vi "ValueSignalLatchBooleanArray.vi"(0 "VI Reference In":refnum<vi>, 5 "Control Path":string[](array[string]), 11 "error in":errorcluster) -> (4 "VI Reference Out":refnum<vi>, 15 "error out":errorcluster)   [LabVIEW 2016, in "Drona.lvlib" / "ControlValue.lvlib"]
doc: "Triggers the latch boolean by keyboard simulation.\n\nThe path of the control should be given in the successive index of the array"
uses:
  ControlValue.lvlib
  KeyBoardSimulation/typedef/VirtualKey.ctl
  VI/MakeVIFrontMost.vi
  Get/GetControlRef/GetControlRef.lvlib
  Drona.lvlib
  KeyBoardSimulation/KeyboardSimulation.lvlib
  VI/VI.lvlib
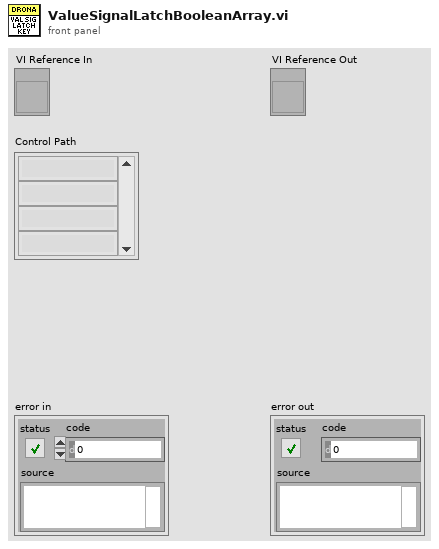
[diagram p1: front panel]
types:
  T1 = typedef "Drona.lvlib/KeyboardSimulation.lvlib/VirtualKey.ctl" = u8
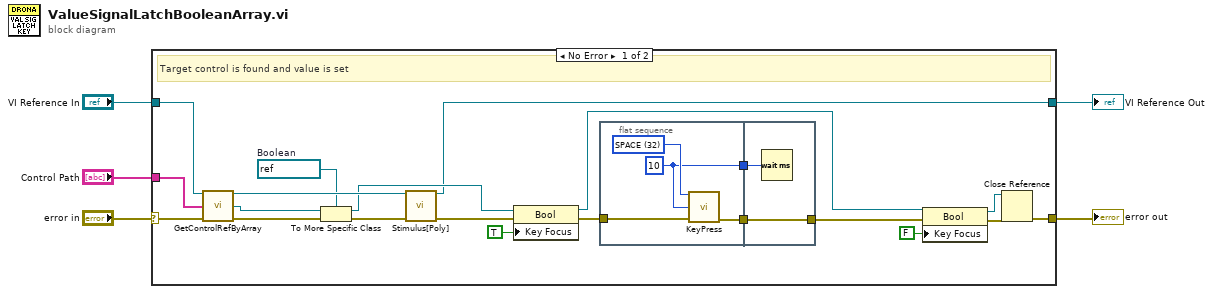
[diagram p0: block diagram]
diagram:
  n1 = case shown="No Error" "error in" {
    selector: "error in" -> [w26 w34]
    tunnel: "Control Path" -> [w24 _]
    tunnel: "VI Reference In" -> [w23 w33]
    tunnel: [w14 w33] -> w2
    tunnel: [w22 w34] -> w1
    frame No Error {
      w18 = refnum<vi> refnum  # Boolean
      # "Target control is found and value is set"
      n2 = call "GetControlRefByArray.vi"("VI Reference In"=w23, "Control Path"=w24, "error In"=w26) -> ("VI Reference Out"=w20:refnum<vi>, "Ctl Refnum"=w21:refnum<vi>, "error out"=w25:errorcluster)  [unwired: 10 in]
      n3 = To More Specific Class(target class=w18, reference=w21, error in=w25) -> (specific class reference=w17:refnum<vi>, error out=w19:errorcluster)
      n4 = call-poly "Stimulus[Poly].vi"("VI Reference In"=w20, "error in"=w19) -> ("VI Reference Out"=w14:refnum<vi>, "error out"=w16:errorcluster)  [unwired: 12 in]
      n5 = property class="Bool"(reference=w17, error in=w16, "Key Focus"=TRUE) -> (reference out=w12:refnum<vi>, error out=w9:errorcluster)
      n6 = flat-sequence {
        tunnel: w9 -> [w30]
        tunnel: [w29] -> w7
        tunnel: [w27] -> w6
        tunnel: [w32] -> w8
        tunnel: w7 -> [w32]
        tunnel: w6 -> [w31]
        frame #0 {
          w27 = u32 10 ("Millis")
          w28 = T1 32 items=["LBUTTON"=1, "RBUTTON"=2, "CANCEL"=3, "MBUTTON"=4, "BACKSPACE"=8, "TAB"=9, "CLEAR"=12, "ENTER"=13, "SHIFT"=16, "CTRL"=17, "ALT"=18, "PAUSE"=19, "CAPITAL"=20, "ESCAPE"=27, "SPACE"=32, "PAGEUP"=33, "PAGEDOWN"=34, "END"=35, "HOME"=36, "LEFTARROW"=37, "UPARROW"=38, "RIGHTARROW"=39, "DOWNARROW"=40, "SELECT"=41, "PRINT"=42, "EXECUTE"=43, "PRINTSCREEN"=44, "INSERT"=45, "DELETE"=46, "HELP"=47, "0"=48, "1"=49, "2"=50, "3"=51, "4"=52, "5"=53, "6"=54, "7"=55, "8"=56, "9"=57, "A"=65, "B"=66, "C"=67, "D"=68, "E"=69, "F"=70, "G"=71, "H"=72, "I"=73, "J"=74, "K"=75, "L"=76, "M"=77, "N"=78, "O"=79, "P"=80, "Q"=81, "R"=82, "S"=83, "T"=84, "U"=85, "V"=86, "W"=87, "X"=88, "Y"=89, "Z"=90, "LWIN"=91, "RWIN"=92, "APPS"=93, "NUMPAD0"=96, "NUMPAD1"=97, "NUMPAD2"=98, "NUMPAD3"=99, "NUMPAD4"=100, "NUMPAD5"=101, "NUMPAD6"=102, "NUMPAD7"=103, "NUMPAD8"=104, "NUMPAD9"=105, "MULTIPLY"=106, "ADD"=107, "SEPERATOR"=108, "SUBTRACT"=109, "DECIMAL"=110, "DIVIDE"=111, "F1"=112, "F2"=113, "F3"=114, "F4"=115, "F5"=116, "F6"=117, "F7"=118, "F8"=119, "F9"=120, "F10"=121, "F11"=122, "F12"=123, "F13"=124, "F14"=125, "F15"=126, "F16"=127, "F17"=128, "F18"=129, "F19"=130, "F20"=131, "F21"=132, "F22"=133, "F23"=134, "F24"=135, "NUMLOCK"=144, "SCROLL"=145, "LSHIFT"=160, "RSHIFT"=161, "LCTRL"=162, "RCTRL"=163, "LALT"=164, "RALT"=165, "VOLMUTE"=173, "VOLDOWN"=174, "VOLUP"=175, ";    :"=186, "=   +"=187, ",    <"=188, "-    _"=189, ".    >"=190, "/    ?"=191, "`    ~"=192, "[    {"=219, "\\    |"=220, "]    }"=221, "'    \""=222] ("Virtual Key")
          n7 = call "KeyPress.vi"("Virtual Key"=w28, "Millis"=w27, "error in"=w30) -> ("error out"=w29:errorcluster)  [unwired: 12 in]
        }
        frame #1 {
          n8 = Wait (ms)(milliseconds to wait=w31) -> ()  [unwired: 1 out]
        }
      }
      n9 = property class="Bool"(reference=w12, error in=w8, "Key Focus"=FALSE) -> (reference out=w11:refnum<vi>, error out=w13:errorcluster)
      n10 = Close Reference(reference=w11, error in (no error)=w13) -> (error out=w22:errorcluster)
    }
    frame Error {
    }
  }
  "error out" <- w1
  "VI Reference Out" <- w2
